vi "test_DiscoveryWrapper_StopDiscoveryService_WrapperMethodsWorkWithoutError.vi"(8 "error in":errorcluster) -> (0 "error out":errorcluster, 2 "result":string, 3 "pass":bool)   [LabVIEW 2020, in "MeasurementServerTests.lvlib" / "Discovery Tests.lvlib"]
uses:
  Discovery Tests.lvlib
  Runtime/MeasurementLink Discovery Client/RPC Messages/ni_measurementlink_discovery_v1_ResolveServiceRequest.ctl
  MeasurementServerTests.lvlib
  Runtime/MeasurementLink Discovery V1/MeasurementLink Discovery V1.lvlib
  Runtime/MeasurementLink Discovery Client/MeasurementLink Discovery Client.lvlib
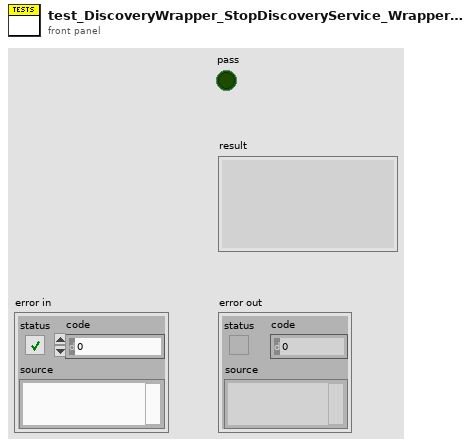
[diagram p1: front panel]
types:
  T1 = typedef "MeasurementLink Discovery Client.lvlib/ni_measurementlink_discovery_v1_ResolveServiceRequest.ctl" = cluster{"provided_interface":string, "service_class":string}
  T2 = typedef "MeasurementLink Discovery Client.lvlib/ni_measurementlink_discovery_v1_ServiceLocation.ctl" = cluster{"location":string, "insecure_port":string, "ssl_authenticated_port":string}
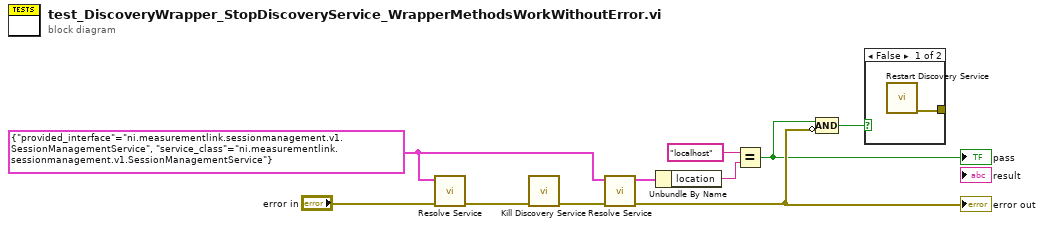
[diagram p0: block diagram]
diagram:
  w2 = T1 {"provided_interface"="ni.measurementlink.sessionmanagement.v1.SessionManagementService", "service_class"="ni.measurementlink.sessionmanagement.v1.SessionManagementService"} ("request data")
  n1 = call "Resolve Service.vi"("error in"="error in", "request data"=w2) -> ("error out"=w1:errorcluster)  [unwired: 8 in, 1 out]
  n2 = call "Kill Discovery Service.vi"("error in"=w1) -> ("error out"=w8:errorcluster)  [unwired: 10 in]
  n3 = call "Resolve Service.vi"("error in"=w8, "request data"=w2) -> ("error out"=w9:errorcluster, "response data"=w7:T2)  [unwired: 8 in]
  "error out" <- w9
  n4 = Unbundle By Name(w7) -> ("location"=w6:string)
  n5 = Equal?(x="localhost", y=w6) -> (x = y?=w5:bool)
  "pass" <- w5
  n6 = Compound Arithmetic op=AND(w5, invert w9) -> (w10:bool)
  n7 = case shown="False" w10 {
    tunnel: [w11 _] -> _
    frame False {
      n8 = call "Restart Discovery Service.vi"() -> ("error out"=w11:errorcluster)  [unwired: 11 in]
    }
    frame True {
    }
  }
